vi "Close skywire serial comm if was opened.vi"(8 "error in (no error)":errorcluster, 10 "Is serial open?":bool, 11 "VISA Refnum in":refnum<visa-resource-name>) -> (0 "error out":errorcluster, 3 "VISA resource name out":refnum<visa-resource-name>)   [LabVIEW 2013]
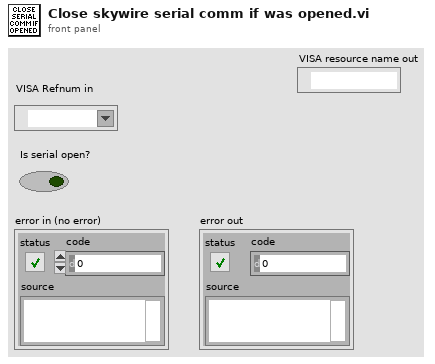
[diagram p1: front panel]
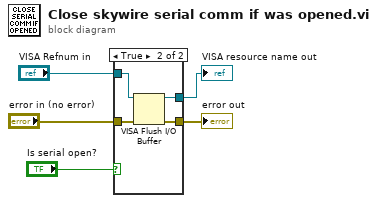
[diagram p0: block diagram]
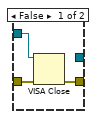
[diagram p2: hidden frame]
diagram:
  n1 = case shown="True" "Is serial open?" {
    tunnel: "error in (no error)" -> [w8 w12]
    tunnel: [w7 w11] -> w3
    tunnel: "VISA Refnum in" -> [w6 w10]
    tunnel: [_ w9] -> w1
    frame False {
      n2 = VISA Close(VISA resource name=w6, error in (no error)=w8) -> (error out=w7:errorcluster)
    }
    frame True {
      n3 = VISA Flush I/O Buffer(VISA resource name=w10, error in (no error)=w12) -> (VISA resource name out=w9:refnum<visa-resource-name>, error out=w11:errorcluster)  [unwired: 1 in]
    }
  }
  "error out" <- w3
  "VISA resource name out" <- w1
